vi "Scan For Projects.vi"(8 "error in (no error)":errorcluster) -> (0 "error out":errorcluster, 3 "Selected Project":refnum<vi>)   [LabVIEW 2014]
panel:
  in  "Open Projects":i32(listbox)
  in  "Cancel":bool
  # "Select An Open Project To Scan"
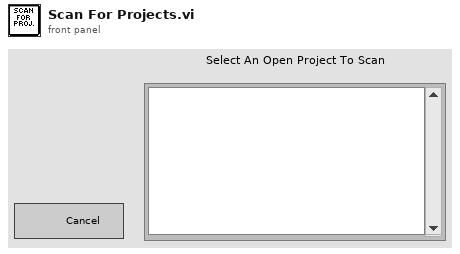
[diagram p1: front panel]
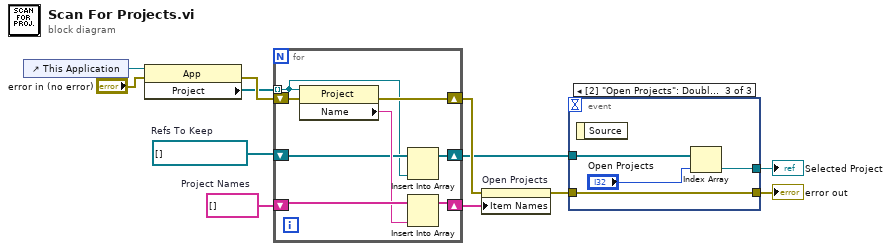
[diagram p0: block diagram]
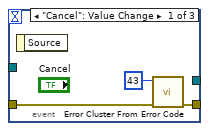
[diagram p2: hidden frame]
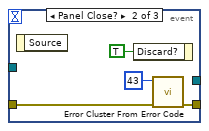
[diagram p3: hidden frame]
diagram:
  w9 = refnum<vi>[] []  # Refs To Keep
  w11 = string[] []  # Project Names
  n1 = control-ref of="This Application"() -> (w8:refnum<vi>)
  n2 = property class="App"(reference=w8, error in="error in (no error)") -> (error out=w12:errorcluster, "Project"=w10:refnum<vi>[])  [unwired: 1 out]
  n3 = for {
    tunnel: w10 -> [w13] mode=indexing
    shift-right: [w19] -> w6
    shift-left: w12 -> [w20]
    shift-right: [w16] -> w7
    shift-left: w11 -> [w18]
    shift-right: [w14] -> w4
    shift-left: w9 -> [w15]
    n4 = property class="Project"(reference=w13, error in=w20) -> (error out=w19:errorcluster, "Name"=w17:string)  [unwired: 1 out]
    n5 = Insert Into Array(array=w15, new element=w13) -> (w14:refnum<vi>[])  [unwired: 1 in]
    n6 = Insert Into Array(array=w18, new element=w17) -> (w16:string[])  [unwired: 1 in]
  }
  n7 = property on="Open Projects" class="LstBox (strict)"(error in=w6, "Item Names"=w7) -> (error out=w5:errorcluster)  [unwired: 1 in, 1 out]
  n8 = event shown="[2] \"Open Projects\": Double Click" {
    selector: _ -> [_ _ _]
    dyn-events: _ -> [_ _ _]
    timeout: _ -> [_ _ _]
    tunnel: w5 -> [w23 w27 w28]
    tunnel: w4 -> [_ _ w31]
    tunnel: [_ _ w29] -> w3
    tunnel: [w22 w26 w28] -> w2
    event "Cancel": Value Change {
      n9 = event-data() -> ()  [unwired: 1 in, 1 out]
      n10 = call <vilib>:"Error Cluster From Error Code.vi"("error in (no error)"=w23, "error code (0)"=43) -> ("error out"=w22:errorcluster)  [unwired: 7 in]
    }
    event Panel Close? {
      n11 = event-data() -> ()  [unwired: 1 in, 1 out]
      n12 = event-data("Discard?"=TRUE) -> ()  [unwired: 1 in, 1 out]
      n13 = call <vilib>:"Error Cluster From Error Code.vi"("error in (no error)"=w27, "error code (0)"=43) -> ("error out"=w26:errorcluster)  [unwired: 7 in]
    }
    event "Open Projects": Double Click {
      n14 = event-data() -> ()  [unwired: 1 in, 1 out]
      n15 = Index Array(array=w31, index="Open Projects") -> (element=w29:refnum<vi>)
    }
  }
  "Selected Project" <- w3
  "error out" <- w2
